vi "Add Foreign Key.vi"(8 "error in (no error)":errorcluster, 9 "FK Info":T1, 10 "Column Name":string, 11 "Table Configuration Basic DB in":refnum<class "Table Configuration Basic DB.lvclass">) -> (0 "error out":errorcluster, 3 "Table Configuration Basic DB out":refnum<class "Table Configuration Basic DB.lvclass">)   [LabVIEW 2020, in "Table.lvlib" / "Table Configuration Basic DB.lvclass"]
uses:
  Table Configuration Basic DB.lvclass
  C:/Users/User/Desktop/Raman Program/Database OOP/source/Database OOP/Table Libraries/Basic Table/Configuration/Table Configuration Class/Table Configuration.lvclass
  Legacy/Field/FK Info.ctl
  Table Configuration Class/Table Configuration.lvclass/Table Configuration.ctl
  Table Configuration Class/Table Configuration.lvclass
  Column Libraries/Column Interfaces.lvlib
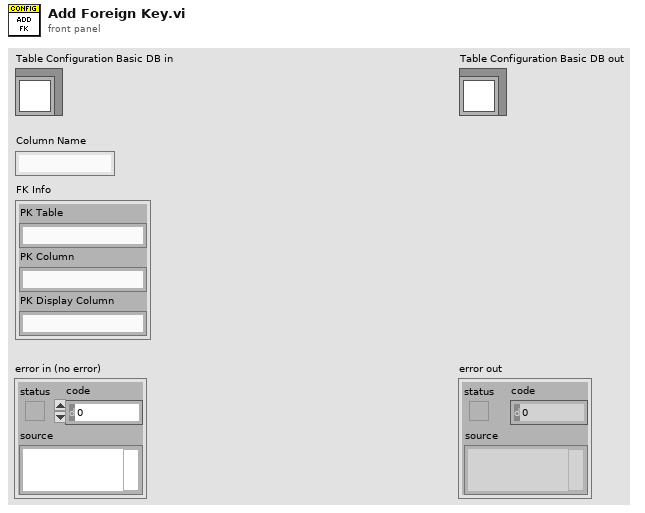
[diagram p1: front panel]
types:
  T1 = typedef "Column Interfaces.lvlib/FK Info.ctl" = cluster{"PK Table":string, "PK Column":string, "PK Display Column":string}
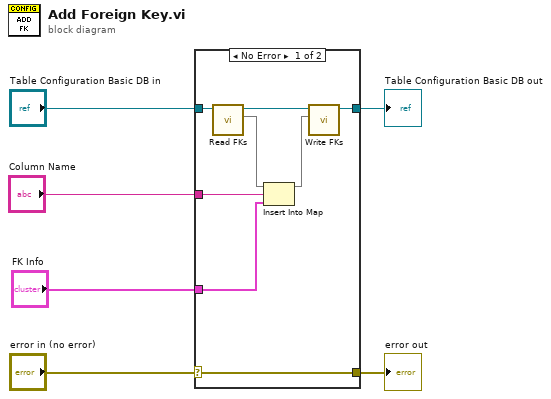
[diagram p0: block diagram]
diagram:
  n1 = case shown="No Error" "error in (no error)" {
    selector: "error in (no error)" -> [w14 w16]
    tunnel: [w14 w16] -> w5
    tunnel: [w13 w15] -> w3
    tunnel: "Table Configuration Basic DB in" -> [w9 w15]
    tunnel: "Column Name" -> [w11 _]
    tunnel: "FK Info" -> [w10 _]
    frame No Error {
      n2 = call "Read FKs.vi"("Table Configuration in"=w9) -> ("FKs"=w7:map{string, T1}, "Table Configuration out"=w8:refnum<class "Table Configuration Basic DB.lvclass">)  [unwired: 8 in, 1 out]
      n3 = Insert Into Map(map in=w7, key=w11, value=w10) -> (map out=w12:map{string, T1})  [unwired: 2 out]
      n4 = call "Write FKs.vi"("FKs"=w12, "Table Configuration in"=w8) -> ("Table Configuration out"=w13:refnum<class "Table Configuration Basic DB.lvclass">)  [unwired: 8 in, 1 out]
    }
    frame Error {
    }
  }
  "error out" <- w5
  "Table Configuration Basic DB out" <- w3
